vi "Read Full Output.vi"(6 "maximal byte count (-1)":i32=-1, 7 "timeout [ms]":u32, 8 "error in":errorcluster, 11 "pipe in":T1) -> (0 "error out":errorcluster, 2 "read buffer":string, 3 "pipe out":T1, 5 "bytes remaining":i32)   [LabVIEW 2013, in "GOLPI library.lvlib"]
doc: "Reads full output of GNU Octave buffered in stdout pipe.\nIf timeout is exceeded, returns only part of buffer and returns number of bytes remaining in the stdout buffer.\nReading also stops if maximal byte count is greater than zero and number of red bytes reaches this limit."
uses:
  GOLPI library.lvlib
  LV Process.lvlibp/Pipe Handle.ctl
  LV Process.lvlibp
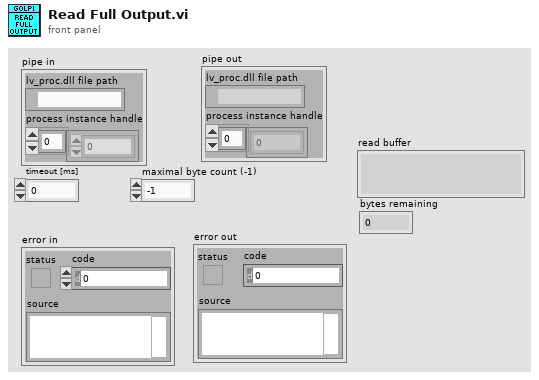
[diagram p1: front panel]
types:
  T1 = typedef "LV Process.lvlibp/Pipe Handle.ctl" = cluster{"lv_proc.dll file path":path, "process instance handle":u32[]}
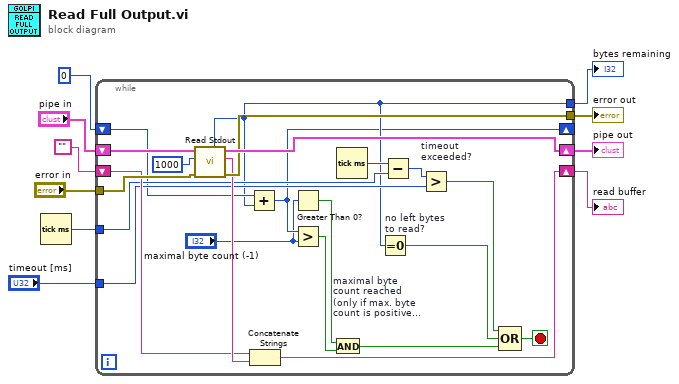
[diagram p0: block diagram]
diagram:
  n1 = Tick Count (ms)() -> (millisecond timer value=w3:u32)
  n2 = while {
    tunnel: [w30] -> w8
    tunnel: "error in" -> [w29]
    tunnel: [w16] -> w5
    shift-right: [w31] -> w9
    shift-left: "pipe in" -> [w32]
    shift-right: [w26] -> w6
    shift-left: "" -> [w27]
    tunnel: w3 -> [w24]
    tunnel: "timeout [ms]" -> [w21]
    shift-right: [w15] -> _
    shift-left: 0 -> [w18]
    stop <- w19 stop-if-true
    n3 = call "Read Stdout.vi"("error in"=w29, "byte count"=1000, "pipe in"=w32) -> ("error out"=w30:errorcluster, "read buffer"=w28:string, "pipe out"=w31:T1, "bytes remaining"=w16:i32)  [unwired: 3 in, 2 out]
    n4 = Add(x=w18, y=w16) -> (x+y=w15:i32)
    n5 = Concatenate Strings(w27, w28) -> (w26:string)
    n6 = Greater Than 0?(x="maximal byte count (-1)") -> (x > 0?=w14:bool)
    n7 = Greater?(x=w15, y="maximal byte count (-1)") -> (0:w12:bool)
    n8 = And "maximal byte\ncount reached\n(only if max. byte\ncount is positive\nand nonzero)?"(x=w14, y=w12) -> (x .and. y?=w11:bool)
    n9 = Tick Count (ms)() -> (millisecond timer value=w25:u32)
    n10 = Equal To 0? "no left bytes\nto read?"(x=w16) -> (x = 0?=w22:bool)
    n11 = Subtract(x=w25, y=w24) -> (x-y=w23:u32)
    n12 = Greater? "timeout\nexceeded?"(x=w23, y=w21) -> (0:w20:bool)
    n13 = Compound Arithmetic op=OR(w20, w22, w11) -> (w19:bool)
  }
  "pipe out" <- w9
  "error out" <- w8
  "read buffer" <- w6
  "bytes remaining" <- w5
